vi "Step_3_Ans_While_loop.vi"   [LabVIEW 2012]
types:
  T1 = typedef "BotSpeak_Control.ctl" = cluster{"Address":string, "Reply EOF":string, "Hardware":string, "Retries":i8, "Timeout":i32}
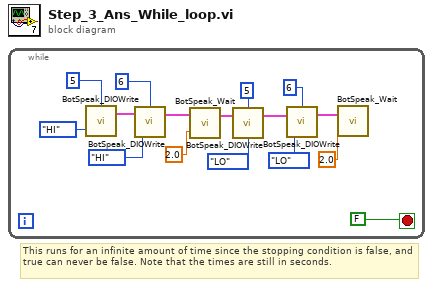
[diagram p0: block diagram]
diagram:
  # "This runs for an infinite amount of time since the stopping condition is false, and true can never be false. Note that the times are still in seconds."
  n1 = while {
    stop <- FALSE stop-if-true
    n2 = call <userlib>:"BotSpeak_DIOWrite.vi"("State"=enum32{"LO", "HI"}."HI", "DIO Line"=u32 5) -> ("Bot Settings"=w14:T1)  [unwired: 1 in, 1 out]
    n3 = call <userlib>:"BotSpeak_DIOWrite.vi"("State"=enum32{"LO", "HI"}."HI", "Bot Settings"=w14, "DIO Line"=u32 6) -> ("Bot Settings"=w11:T1)  [unwired: 1 out]
    n4 = call <userlib>:"BotSpeak_Wait.vi"("Wait (sec)"=2.0, "Bot Settings"=w11) -> ("Bot Settings"=w4:T1)  [unwired: 1 in]
    n5 = call <userlib>:"BotSpeak_DIOWrite.vi"("State"=enum32{"LO", "HI"}."LO", "Bot Settings"=w4, "DIO Line"=u32 5) -> ("Bot Settings"=w7:T1)  [unwired: 1 out]
    n6 = call <userlib>:"BotSpeak_DIOWrite.vi"("State"=enum32{"LO", "HI"}."LO", "Bot Settings"=w7, "DIO Line"=u32 6) -> ("Bot Settings"=w3:T1)  [unwired: 1 out]
    n7 = call <userlib>:"BotSpeak_Wait.vi"("Wait (sec)"=2.0, "Bot Settings"=w3) -> ()  [unwired: 1 in, 1 out]
  }
